vi "channel_signal.vi"() -> ()   [LabVIEW 2017]
doc: "Illustrates how to send a signal to a long-running process on a SSH server."
uses:
  libssh2/libssh2_session_handshake_tcp.vi
  libssh2/Wait Socket (TCP).vi
  libssh2/libssh2_init_default.vi
  libssh2/libssh2_session_init_ex.vi
  <vilib>/Utility/tcp.llb/TCP Get Raw Net Object.vi
  libssh2/libssh2_session_handshake_socket.vi
  libssh2/libssh2_userauth_password_ex.vi
  libssh2/libssh2_channel_open_ex.vi
  libssh2/libssh2_channel_process_startup.vi
  libssh2/Wait Socket (Socket).vi
  libssh2/libssh2_channel_read_ex.vi
  libssh2/libssh2.lvlib
panel:
  in  "Terminate":bool
  out "read buffer":string
  in  "password":string
  in  "username":string
  in  "hostname":string="localhost"
  out "error out":errorcluster
  # "Continuously runs a \"ping\" command on\nthe SSH server until it is terminated by the\nuser."
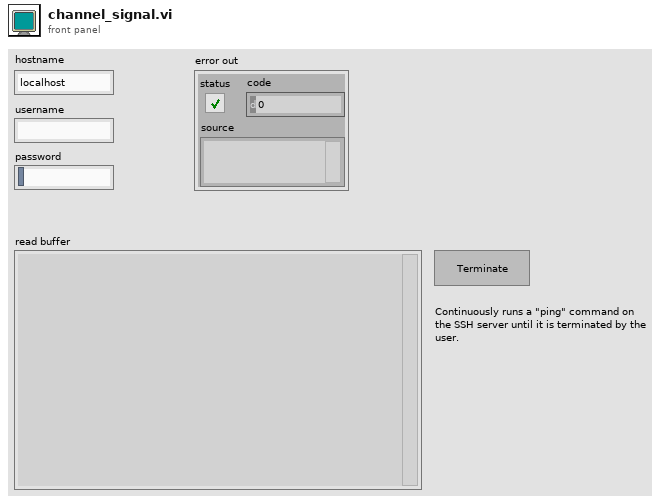
[diagram p1: front panel]
types:
  T1 = typedef "libssh2.lvlib/Session Refnum.ctl" = refnum<k1>
  T2 = typedef "libssh2.lvlib/Channel Refnum.ctl" = refnum<k1>
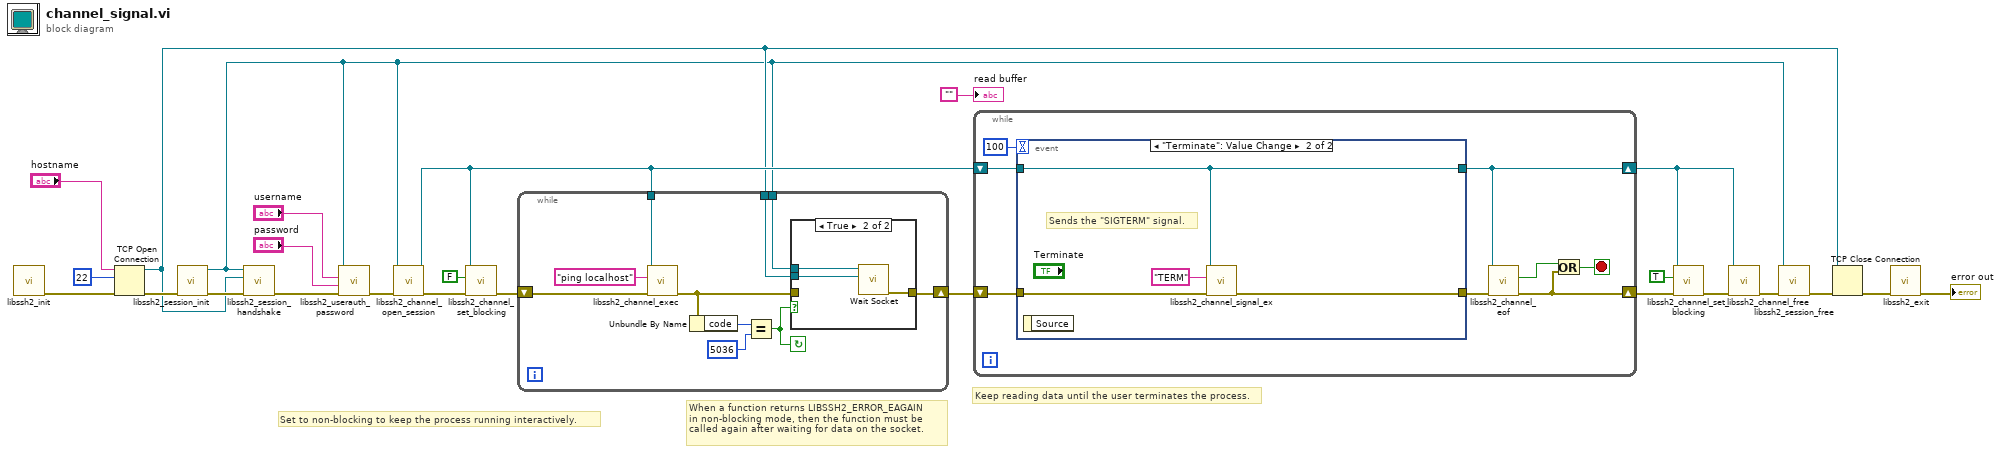
[diagram p0: block diagram]
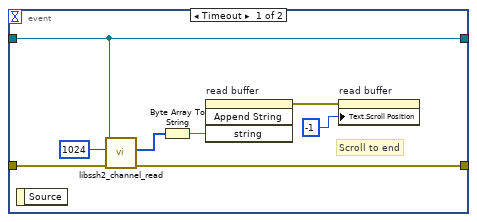
[diagram p3: hidden frame]
diagram:
  # "Keep reading data until the user terminates the process."
  # "When a function returns LIBSSH2_ERROR_EAGAIN\nin non-blocking mode, then the function must be\ncalled again after waiting for data on the socket."
  # "Set to non-blocking to keep the process running interactively."
  n1 = call-poly "libssh2_init.vi"() -> ("error out"=w25:errorcluster)  [unwired: 11 in]
  n2 = TCP Open Connection(address="hostname", remote port or service name=u16 22, error in (no error)=w25) -> (connection ID=w3:refnum<k5>, error out=w7:errorcluster)  [unwired: 2 in]
  n3 = call "libssh2_session_init.vi"("error in (no error)"=w7) -> ("error out"=w20:errorcluster, "session"=w2:T1)  [unwired: 9 in]
  n4 = call-poly "libssh2_session_handshake.vi"("error in (no error)"=w20, "tcp connection"=w3, "session"=w2) -> ("error out"=w19:errorcluster)  [unwired: 8 in]
  n5 = call "libssh2_userauth_password.vi"("error in (no error)"=w19, "password"="password", "username"="username", "session"=w2) -> ("error out"=w18:errorcluster)  [unwired: 7 in]
  n6 = call "libssh2_channel_open_session.vi"("error in (no error)"=w18, "session"=w2) -> ("error out"=w15:errorcluster, "channel"=w6:T2)  [unwired: 8 in]
  n7 = call "libssh2_channel_set_blocking.vi"("error in (no error)"=w15, "blocking"=FALSE, "channel"=w6) -> ("error out"=w12:errorcluster)  [unwired: 8 in]
  n8 = while {
    tunnel: w6 -> [w33]
    shift-right: [w29] -> w4
    shift-left: w12 -> [w35]
    tunnel: w3 -> [w27]
    tunnel: w2 -> [w26]
    stop <- w30 continue-if-true
    n9 = call "libssh2_channel_exec.vi"("error in (no error)"=w35, "command"="ping localhost", "channel"=w33) -> ("error out"=w28:errorcluster)  [unwired: 8 in]
    n10 = Unbundle By Name(w28) -> ("code"=w32:i32)
    n11 = Equal?(x=w32, y=5036) -> (x = y?=w30:bool)
    n12 = case shown="True" w30 {
      tunnel: [w36 w39] -> w29
      tunnel: w28 -> [w36 _]
      tunnel: w27 -> [_ w37]
      tunnel: w26 -> [_ w38]
      frame False {
      }
      frame True {
        n13 = call-poly "Wait Socket.vi"("tcp connection"=w37, "session"=w38) -> ("error out"=w39:errorcluster)  [unwired: 9 in]
      }
    }
  }
  n14 = while {
    shift-right: [w40] -> w5
    shift-left: w6 -> [w44]
    shift-right: [w46] -> w8
    shift-left: w4 -> [w43]
    stop <- w47 stop-if-true
    n15 = event shown="[1] \"Terminate\": Value Change" {
      selector: _ -> [_ _]
      dyn-events: _ -> [_ _]
      timeout: 100 -> [_ _]
      tunnel: w44 -> [w54 w58]
      tunnel: w43 -> [w53 w56]
      tunnel: [w52 w57] -> w42
      tunnel: [w54 w58] -> w40
      event Timeout {
        # "Scroll to end"
        n16 = event-data() -> ()  [unwired: 1 in, 1 out]
        n17 = call "libssh2_channel_read.vi"("error in (no error)"=w53, "buffer length"=1024, "channel"=w54) -> ("error out"=w52:errorcluster, "buffer"=w51:u8[])  [unwired: 7 in]
        n18 = Byte Array To String(unsigned byte array=w51) -> (string=w50:string)
        n19 = invoke on="read buffer" class="Str" method="Append String"("string"=w50) -> (error out=w48:errorcluster)  [unwired: 3 in, 3 out]
        n20 = property on="read buffer" class="Str"(error in=w48, "Text.Scroll Position"=-1) -> ()  [unwired: 1 in, 2 out]
      }
      event "Terminate": Value Change {
        # "Sends the \"SIGTERM\" signal."
        n21 = event-data() -> ()  [unwired: 1 in, 1 out]
        n22 = call "libssh2_channel_signal_ex.vi"("error in (no error)"=w56, "signal name"="TERM", "channel"=w58) -> ("error out"=w57:errorcluster)  [unwired: 8 in]
      }
    }
    n23 = call "libssh2_channel_eof.vi"("error in (no error)"=w42, "channel"=w40) -> ("error out"=w46:errorcluster, "eof"=w45:bool)  [unwired: 8 in]
    n24 = Or(x=w45, y=w46) -> (x .or. y?=w47:bool)
  }
  n25 = call "libssh2_channel_set_blocking.vi"("error in (no error)"=w8, "blocking"=TRUE, "channel"=w5) -> ("error out"=w10:errorcluster)  [unwired: 8 in]
  n26 = call "libssh2_channel_free.vi"("error in (no error)"=w10, "channel"=w5) -> ("error out"=w13:errorcluster)  [unwired: 9 in]
  n27 = call "libssh2_session_free.vi"("error in (no error)"=w13, "session"=w2) -> ("error out"=w14:errorcluster)  [unwired: 9 in]
  n28 = TCP Close Connection(connection ID=w3, error in (no error)=w14) -> (error out=w22:errorcluster)  [unwired: 1 in, 1 out]
  n29 = call "libssh2_exit.vi"("error in (no error)"=w22) -> ("error out"=→"error out":errorcluster)  [unwired: 10 in]
  "read buffer" <- ""
